vi "grabber fpga details panel.vi"() -> ()   [LabVIEW 2010]
uses:
  scan_specification_tagResonant.ctl
  common_typedefs/DAC_voltage_tagResonantr.ctl
  FPGA_ref.ctl
  <vilib>/Platform/TimedLoop/XDataNode/XDataNode.xnode
  <vilib>/Platform/TimedLoop/XDataNode/timing_clust.ctl
  <vilib>/Platform/TimedLoop/XDataNode/nitl_modes.ctl
  <vilib>/Platform/TimedLoop/XDataNode/wakeup.ctl
  <vilib>/rvi/interface/nirviReadWriteControl/nirviReadWriteControl.xnode
  <vilib>/rvi/interface/common/niFpgaNodeNameForErrorReporting.ctl
  <vilib>/rvi/errors/niLvFpgaWhatHappensToTopLevelVI.ctl
  <vilib>/Utility/error.llb/Error Cluster From Error Code.vi
  <vilib>/rvi/errors/niLvFpgaAdjustHostInterfaceError.vi
  <vilib>/Platform/TimedLoop/XDataNode/XDNodeRunTimeDep.lvlib
  NiFpgaLv.dll
panel:
  out "N spot tracker out":T1
  out "Spot locations":T2(array[cluster])
  out "stim time on":dbl
  out "stim photon rate":dbl format="%#_3p"
  out "y-offset(mv)":dbl
  out "x-offset (mv)":dbl
  out "y-offset":i16
  out "x-offset":i16
  out "z-location":i16
  out "piezo z-offset":i16
  out "piezo out":i16
  in  "FPGARef":T3
  out "scanning? FPGA":bool
  out "scan":bool
  out "FIFO overflow":bool
  out "DAC voltages":T4 {"pockels" max=4095 step=1; "y" max=4095 step=1; "x" max=4095 step=1}
  out "scan specification":T5={"z resolution (pixels)"=100, "iterations per pixel"=28, "iterations per z-scan (=zres*iterperpixel)"=50, "x resolution (pixels)"=100, "y resolution (pixels)"=80, "number of z-lines per volume"=30, "number of repetitions (volumes)"=5, "Pockels cell voltage (bits)"=80, "Vx center (bits)"=0, "Vy center (bits)"=0, "Vx amplitude (bits)"=40, "Vy amplitude (bits)"=0, "lines to delay between scan start and output"=1, "LSB has acquire control"=FALSE, "Pockels cell bleach voltage"=0}
  out "lines sent":u32
  out "pixels sent":u32
  in  "stop":bool
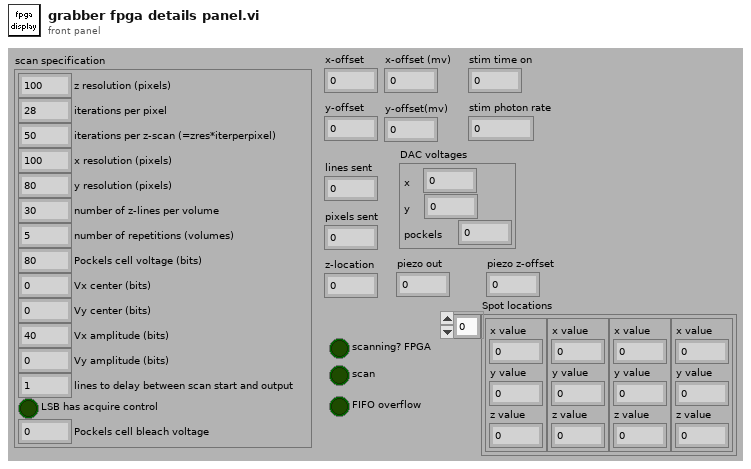
[diagram p1: front panel]
types:
  T1 = cluster{"current state":u8, "number of spots":u8, "circles per spot":u16, "inter-spot delay":u8, "circle counter":u16, "delay counter":u8}
  T2 = cluster{"x value":i16, "y value":i16, "z value":i16}[]
  T3 = typedef "FPGA_ref.ctl" = refnum<k20>
  T4 = typedef "DAC_voltage_tagResonantr.ctl" = cluster{"x":i16, "y":i16, "pockels":i16}
  T5 = typedef "scan_specification_tagResonant.ctl" = cluster{"z resolution (pixels)":u16, "iterations per pixel":u16, "iterations per z-scan (=zres*iterperpixel)":u16, "x resolution (pixels)":u16, "y resolution (pixels)":u16, "number of z-lines per volume":u16, "number of repetitions (volumes)":i32, "Pockels cell voltage (bits)":i16, "Vx center (bits)":i16, "Vy center (bits)":i16, "Vx amplitude (bits)":i16, "Vy amplitude (bits)":i16, "lines to delay between scan start and output":u16, "LSB has acquire control":bool, "Pockels cell bleach voltage":i16}
  T6 = typedef "XDNodeRunTimeDep.lvlib/timing_clust.ctl" = cluster{"Expected End [f-1]":u64, "Actual End [f-1]":u64, "Finished Late? [f-1]":bool, "Expected End [i-1]":u64, "Actual End [i-1]":u64, "Finished Late? [i-1]":bool, "Expected Start [i]":u64, "Actual Start [i]":u64, "Expected Start [f]":u64, "Actual Start [f]":u64, "Source Name":string, "Structure Name":string, "Period":i64, "Deadline":i64, "Offset":i64, "Start":i64, "Priority":i32, "Timeout":i32, "Mode":T7, "Wakeup Reason":T8, "Error":errorcluster, "Source Type":string, "Secondary Source Type":string, "Global End Time":u64, "Global Start Time":u64, "Frame Duration":u64, "Iteration Duration":u64, "Assigned CPU":i32, "I/O Scan Engine Mode":u32}
  T7 = typedef "XDNodeRunTimeDep.lvlib/nitl_modes.ctl" = enum32{"No Change", "Process missed periods, maintain original phase", "Discard missed periods, maintain original phase", "Process missed periods, ignore original phase", "Discard missed periods, ignore original phase"}
  T8 = typedef "XDNodeRunTimeDep.lvlib/wakeup.ctl" = enum32{"Normal", "Aborted", "Asynchronous wakeup", "Timing source error", "Timed loop error", "Timeout"}
  T9 = cluster{"z resolution (pixels)":u16, "iterations per pixel":u16, "iterations per z-scan (=zres*iterperpixel)":u16, "x resolution (pixels)":u16, "y resolution (pixels)":u16, "number of z-lines per volume":u16, "number of repetitions (volumes)":i32, "Pockels cell voltage (bits)":i16, "Vx center (bits)":i16, "Vy center (bits)":i16, "Vx amplitude (bits)":i16, "Vy amplitude (bits)":i16, "lines to delay between scan start and output":u16, "LSB has acquire control":bool, "Pockels cell bleach voltage":i16}
  T10 = typedef "niFpgaNodeNameForErrorReporting.ctl" = enum16{"Open FPGA VI Reference", "Read/Write Control", "Invoke Method: Abort", "Invoke Method: Acknowledge IRQ", "Invoke Method: Download", "Invoke Method: FIFO.Configure", "Invoke Method: FIFO.Read", "Invoke Method: FIFO.Start", "Invoke Method: FIFO.Stop", "Invoke Method: FIFO.Write", "Invoke Method: Reset", "Invoke Method: Run", "Invoke Method: Wait on IRQ", "Close FPGA VI Reference"}
  T11 = typedef "niLvFpgaWhatHappensToTopLevelVI.ctl" = enum16{"top level VI scripted behind XNode", "top level VI inlined behind XNode"}
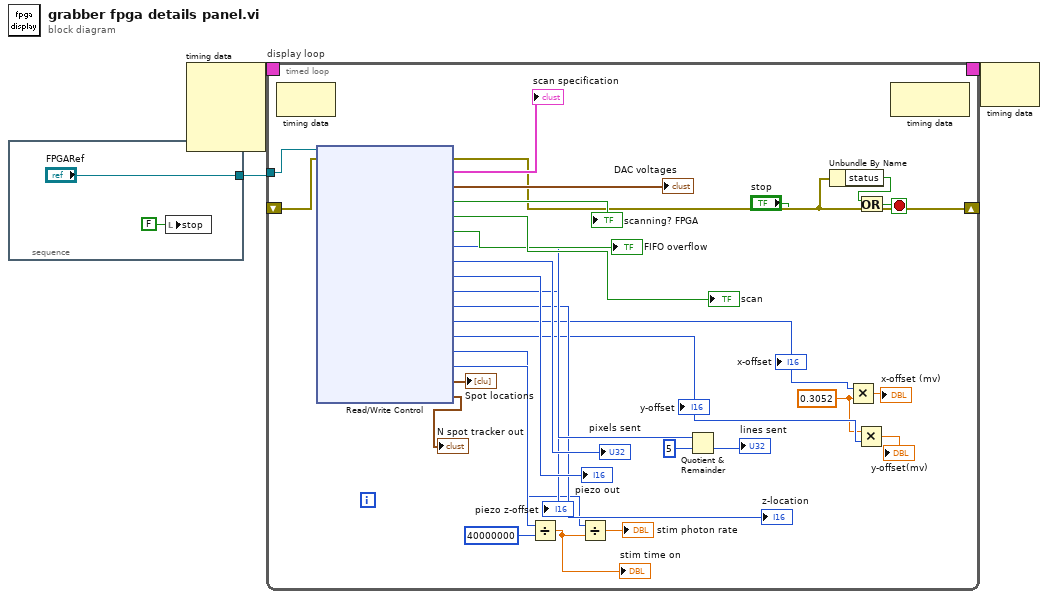
[diagram p0: block diagram]
diagram:
  n1 = stacked-sequence {
    tunnel: ["FPGARef"] -> w1
    frame #0 {
      n2 = local write "stop"(FALSE ("stop")) -> ()
    }
  }
  n3 = node-c288() -> (w3:T6)  [unwired: 4 in]
  n4 = timed-loop "display loop" {
    shift-right: [w24] -> _
    shift-left: _ -> [w25]
    timing: w3 -> [_]
    timing-out: [_] -> w2
    tunnel: w1 -> [w26]
    stop <- w35 stop-if-true
    w14 = 0.3052 ("y")
    n5 = node-c288() -> ()  [unwired: 1 in, 1 out]
    n6 = xnode "Read/Write Control"("FPGA VI Reference In"=w26, "error in"=w25) -> ("error out"=w24:errorcluster, "scan specification"=→"scan specification":T9, "DAC voltages"=→"DAC voltages":cluster{"x":i16, "y":i16, "pockels":i16}, "scanning?"=→"scanning? FPGA":bool, "scan"=→"scan":bool, "FIFO overflow"=→"FIFO overflow":bool, "lines sent"=w29:u32, "pixels sent"=→"pixels sent":u32, "piezo out"=→"piezo out":i16, "piezo z-offset"=→"piezo z-offset":i16, "z-location"=→"z-location":i16, "x-offset"=w17:i16, "y-offset"=w15:i16, "n photons during stim"=w9:u32, "stim time"=w12:u32, "Spot locations"=→"Spot locations":T2, "N spot tracker out"=→"N spot tracker out":T1)  [unwired: 1 out]
    "x-offset" <- w17
    "y-offset" <- w15
    n7 = Divide(x=w12, y=u32 40000000) -> (x/y=w10:dbl)
    "stim time on" <- w10
    n8 = Divide(x=w9, y=w10) -> (x/y=→"stim photon rate":dbl)
    n9 = Quotient & Remainder(x=w29, y=u32 5) -> (floor(x/y)=→"lines sent":u32)  [unwired: 1 out]
    n10 = Unbundle By Name(w24) -> ("status"=w23:bool)
    n11 = Multiply(x=w17, y=w14) -> (x*y=→"x-offset (mv)":dbl)
    n12 = Multiply(x=w14, y=w15) -> (x*y=→"y-offset(mv)":dbl)
    n13 = Or(x=w23, y="stop") -> (x .or. y?=w35:bool)
    n14 = node-c288() -> ()  [unwired: 1 in, 1 out]
  }
  n15 = node-c288(w2) -> ()  [unwired: 1 out]
